vi "RSZVB Trace Delete.vi"(8 "error in (no error)":errorcluster {"code" format="%.0x"}, 9 "Trace Name (Trc1)":string="Trc1", 10 "Channel (1)":i32=1, 11 "VISA session":refnum<visa-resource-name>) -> (0 "error out":errorcluster {"code" format="%.0x"}, 3 "dup VISA session":refnum<visa-resource-name>)   [LabVIEW 2011]
doc: "This VI deletes a trace with a specified trace name and channel.\n\nRemote-control command(s):\nCALCulate<Ch>:PARameter:DELete '<string>'"
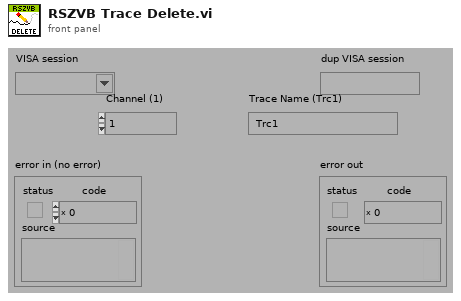
[diagram p1: front panel]
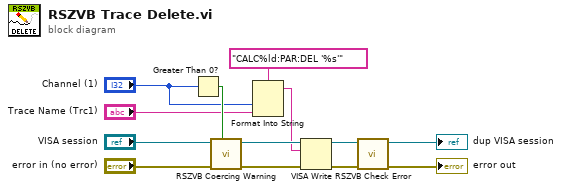
[diagram p0: block diagram]
diagram:
  n1 = Greater Than 0?(x="Channel (1)") -> (x > 0?=w7:bool)
  n2 = call "RSZVB Coercing Warning.vi"("In Range?"=w7, "error in (no error)"="error in (no error)", "VISA session"="VISA session") -> ("error out"=w11:errorcluster, "dup VISA session"=w12:refnum<visa-resource-name>)  [unwired: 7 in]
  n3 = Format Into String(format string="CALC%ld:PAR:DEL '%s'", "Channel (1)", "Trace Name (Trc1)") -> (resulting string=w8:string)  [unwired: 2 in, 1 out]
  n4 = VISA Write(VISA resource name=w12, write buffer=w8, error in (no error)=w11) -> (VISA resource name out=w9:refnum<visa-resource-name>, error out=w10:errorcluster)  [unwired: 1 out]
  n5 = call "RSZVB Check Error.vi"("error in (no error)"=w10, "VISA session"=w9) -> ("error out"=→"error out":errorcluster, "dup VISA session"=→"dup VISA session":refnum<visa-resource-name>)  [unwired: 8 in]
